vi "Offset Inline Buffers.vi"(8 "error in (no error)":errorcluster, 10 "Framework Inline Buffer":refnum<class "Buffer.lvclass">, 11 "Plugin in":refnum<class "Plugin.lvclass">) -> (0 "error out":errorcluster, 3 "Plugin out":refnum<class "Plugin.lvclass">)   [LabVIEW 2017, in "DSF Core.lvlib" / "Plugin.lvclass"]
uses:
  Plugin.lvclass
  Buffer/Buffer.lvclass
  Plugin.lvclass/Plugin.ctl
  Buffers/Buffers.lvclass
  Transfer Group/Transfer Group.lvclass
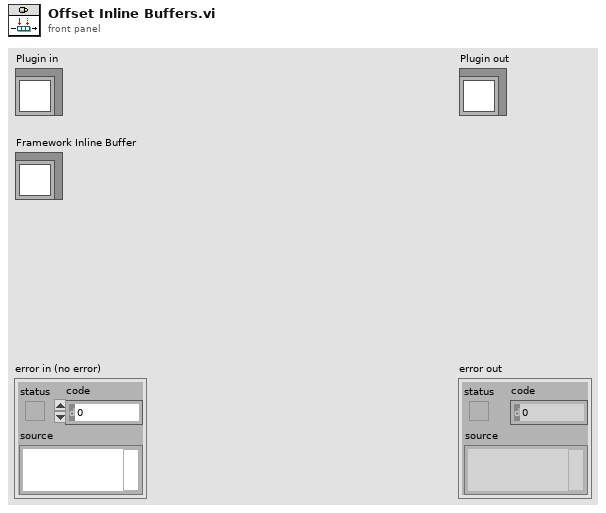
[diagram p1: front panel]
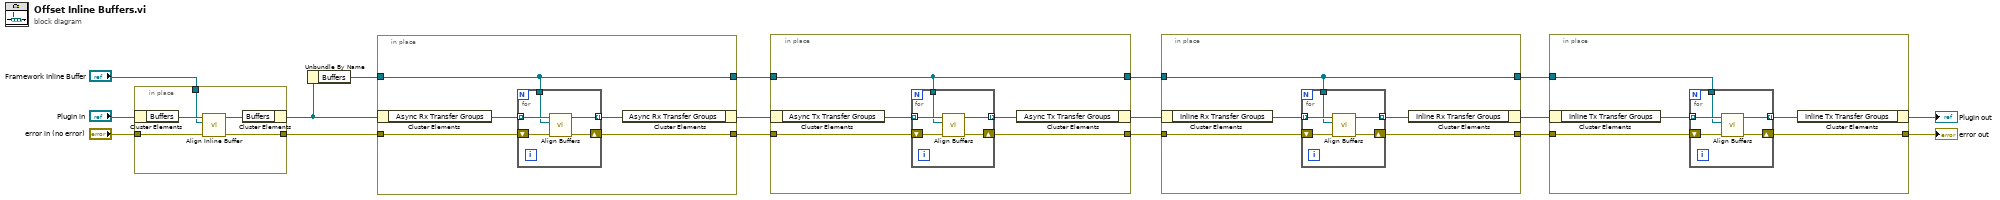
[diagram p0: block diagram]
diagram:
  n1 = in-place {
    in-place-border: "error in (no error)" -> [w21]
    in-place-border: [w19] -> w4
    in-place-border: "Framework Inline Buffer" -> [w18]
    n2 = in-place-cluster #1("Plugin in") -> ("Buffers"=w22:refnum<class "Buffers.lvclass">)
    n3 = call "Align Inline Buffer.vi"("error in (no error)"=w21, "base Inline Buffer"=w18, "Buffers in"=w22) -> ("error out"=w19:errorcluster, "Buffers out"=w20:refnum<class "Buffers.lvclass">)  [unwired: 7 in]
    n4 = in-place-cluster #1("Buffers"=w20) -> (w2:refnum<class "Plugin.lvclass">)
  }
  n5 = Unbundle By Name(w2) -> ("Buffers"=w1:refnum<class "Buffers.lvclass">)
  n6 = in-place {
    in-place-border: w4 -> [w25]
    in-place-border: [w24] -> w16
    in-place-border: [w23] -> w15
    in-place-border: w1 -> [w23]
    n7 = in-place-cluster #2(w2) -> ("Async Rx Transfer Groups"=w27:refnum<class "Transfer Group.lvclass">[])
    n8 = for {
      tunnel: w27 -> [w32] mode=indexing
      tunnel: [w31] -> w26 mode=indexing
      shift-right: [w30] -> w24
      shift-left: w25 -> [w29]
      tunnel: w23 -> [w28]
      n9 = call "Align Buffers.vi"("error in (no error)"=w29, "Plugin Buffers"=w28, "Transfer Group in"=w32) -> ("error out"=w30:errorcluster, "Transfer Group out"=w31:refnum<class "Transfer Group.lvclass">)  [unwired: 7 in]
    }
    n10 = in-place-cluster #2("Async Rx Transfer Groups"=w26) -> (w17:refnum<class "Plugin.lvclass">)
  }
  n11 = in-place {
    in-place-border: w16 -> [w35]
    in-place-border: w15 -> [w33]
    in-place-border: [w34] -> w13
    in-place-border: [w33] -> w12
    n12 = in-place-cluster #3(w17) -> ("Async Tx Transfer Groups"=w37:refnum<class "Transfer Group.lvclass">[])
    n13 = for {
      tunnel: w37 -> [w42] mode=indexing
      tunnel: [w41] -> w36 mode=indexing
      shift-right: [w40] -> w34
      shift-left: w35 -> [w39]
      tunnel: w33 -> [w38]
      n14 = call "Align Buffers.vi"("error in (no error)"=w39, "Plugin Buffers"=w38, "Transfer Group in"=w42) -> ("error out"=w40:errorcluster, "Transfer Group out"=w41:refnum<class "Transfer Group.lvclass">)  [unwired: 7 in]
    }
    n15 = in-place-cluster #3("Async Tx Transfer Groups"=w36) -> (w14:refnum<class "Plugin.lvclass">)
  }
  n16 = in-place {
    in-place-border: w13 -> [w45]
    in-place-border: w12 -> [w43]
    in-place-border: [w44] -> w10
    in-place-border: [w43] -> w9
    n17 = in-place-cluster #4(w14) -> ("Inline Rx Transfer Groups"=w47:refnum<class "Transfer Group.lvclass">[])
    n18 = for {
      tunnel: w47 -> [w52] mode=indexing
      tunnel: [w51] -> w46 mode=indexing
      shift-right: [w50] -> w44
      shift-left: w45 -> [w49]
      tunnel: w43 -> [w48]
      n19 = call "Align Buffers.vi"("error in (no error)"=w49, "Plugin Buffers"=w48, "Transfer Group in"=w52) -> ("error out"=w50:errorcluster, "Transfer Group out"=w51:refnum<class "Transfer Group.lvclass">)  [unwired: 7 in]
    }
    n20 = in-place-cluster #4("Inline Rx Transfer Groups"=w46) -> (w11:refnum<class "Plugin.lvclass">)
  }
  n21 = in-place {
    in-place-border: w10 -> [w54]
    in-place-border: w9 -> [w55]
    in-place-border: [w53] -> w7
    n22 = in-place-cluster #5(w11) -> ("Inline Tx Transfer Groups"=w57:refnum<class "Transfer Group.lvclass">[])
    n23 = for {
      tunnel: w57 -> [w62] mode=indexing
      tunnel: [w61] -> w56 mode=indexing
      shift-right: [w60] -> w53
      shift-left: w54 -> [w59]
      tunnel: w55 -> [w58]
      n24 = call "Align Buffers.vi"("error in (no error)"=w59, "Plugin Buffers"=w58, "Transfer Group in"=w62) -> ("error out"=w60:errorcluster, "Transfer Group out"=w61:refnum<class "Transfer Group.lvclass">)  [unwired: 7 in]
    }
    n25 = in-place-cluster #5("Inline Tx Transfer Groups"=w56) -> (→"Plugin out":refnum<class "Plugin.lvclass">)
  }
  "error out" <- w7
